vi "FGV - Acquisition Status.vi"(7 "Actions":T3=enum."Clear", 8 "Error In":errorcluster, 9 "Hardware in":T1, 10 "Scan Type [In]":T2, 11 "Status In":bool) -> (0 "Error Out":errorcluster, 1 "Hardware out":T1, 2 "Scan Type [Out]":T2, 3 "Status Out":bool)   [LabVIEW 2018]
uses:
  Controls/FGV Actions.ctl
  Controls/ScanType.ctl
  Controls/Hardware control.ctl
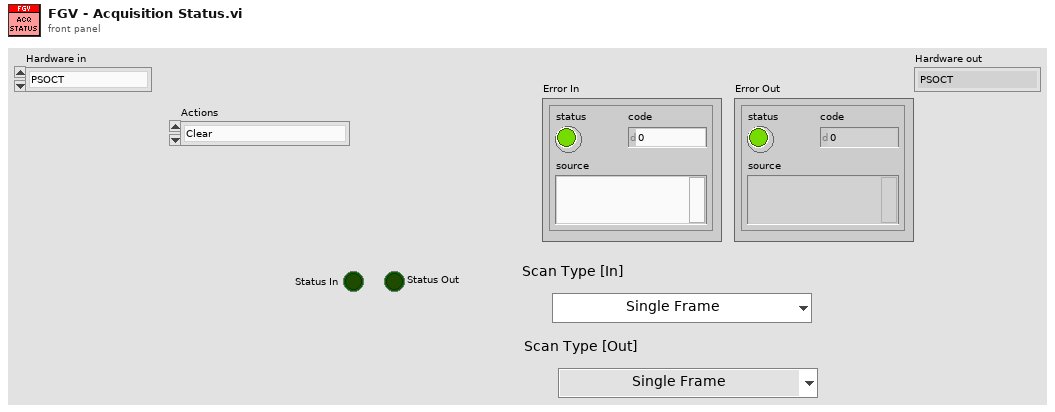
[diagram p1: front panel]
types:
  T1 = typedef "Hardware control.ctl" = enum16{"PSOCT", "Thorlabs OCT"}
  T2 = typedef "ScanType.ctl" = enum16{"Single Frame", "Continuous Frame", "ROI Line", "Vibratome", "Mosaic", "Mosaic + Slice"}
  T3 = typedef "FGV Actions.ctl" = enum16{"Init", "Set", "Get", "Clear"}
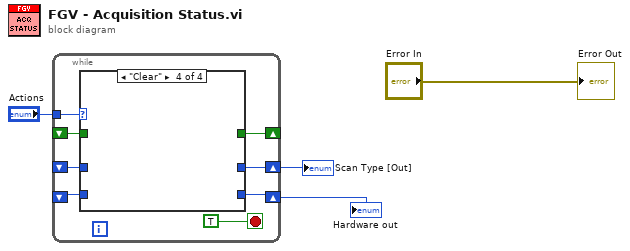
[diagram p0: block diagram]
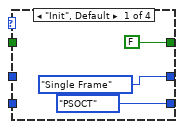
[diagram p2: hidden frame]
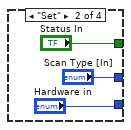
[diagram p3: hidden frame]
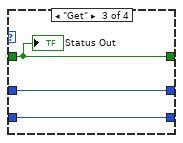
[diagram p4: hidden frame]
diagram:
  n1 = while {
    tunnel: "Actions" -> [w11]
    shift-right: [w10] -> _
    shift-left: _ -> [w9]
    shift-right: [w8] -> w2
    shift-left: _ -> [w7]
    shift-right: [w6] -> w1
    shift-left: _ -> [w5]
    stop <- TRUE stop-if-true
    n2 = case shown="\"Clear\"" w11 {
      tunnel: [FALSE "Status In" w21 _] -> w10
      tunnel: w9 -> [_ _ w21 _]
      tunnel: [ScanType."Single Frame" ("Scan Type") "Scan Type [In]" w20 _] -> w8
      tunnel: w7 -> [_ _ w20 _]
      tunnel: [Hardware_control."PSOCT" "Hardware in" w19 _] -> w6
      tunnel: w5 -> [_ _ w19 _]
      frame "Init", Default {
      }
      frame "Set" {
      }
      frame "Get" {
        "Status Out" <- w21
      }
      frame "Clear" {
      }
    }
  }
  "Scan Type [Out]" <- w2
  "Hardware out" <- w1
  "Error Out" <- "Error In"
